vi "StringifiedData.vi"(8 "error in (no error)":errorcluster, 11 "DoubleArrayMsg in":refnum<class "DoubleArrayMsg.lvclass">) -> (0 "error out":errorcluster, 2 "Stringified Data":string, 3 "DoubleArrayMsg out":refnum<class "DoubleArrayMsg.lvclass">)   [LabVIEW 2018, in "LapDog.Messaging.v3.NativeArrays.lvlib" / "DoubleArrayMsg.lvclass"]
doc: "This VI is used for the message probe. Child classes may override it and provide the message data in string format or a short string describing the data the message contains. This string will be displayed in the probe window."
uses:
  DoubleArrayMsg.lvclass
  DoubleArrayMsg.lvclass/DoubleArrayMsg.ctl
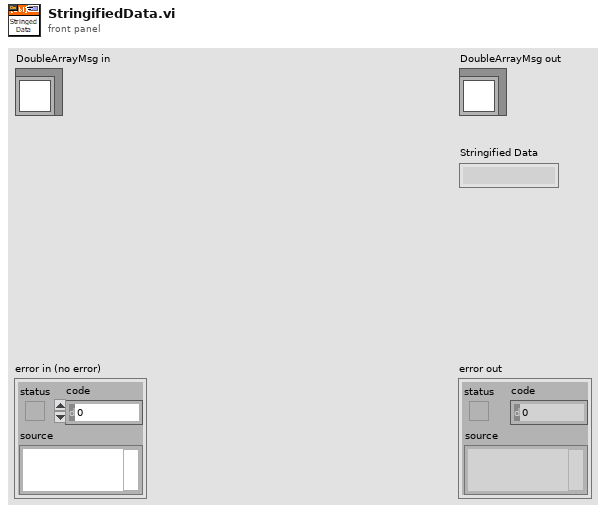
[diagram p1: front panel]
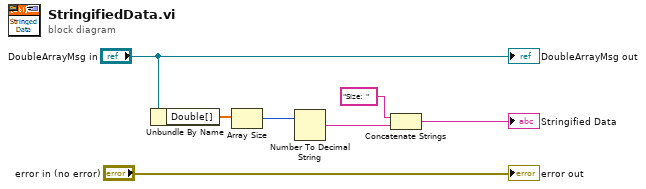
[diagram p0: block diagram]
diagram:
  n1 = Unbundle By Name("DoubleArrayMsg in") -> ("Double[]"=w1:dbl[])
  n2 = Array Size(array=w1) -> (size(s)=w6:i32)
  n3 = Number To Decimal String(number=w6) -> (decimal integer string=w4:string)  [unwired: 1 in]
  n4 = Concatenate Strings("Size:  " ("string"), w4) -> (→"Stringified Data":string)
  "error out" <- "error in (no error)"
  "DoubleArrayMsg out" <- "DoubleArrayMsg in"
